vi "Autonomous selections.vi"() -> (3 "Autonomous selections":string[](array[string]))   [LabVIEW 2015]
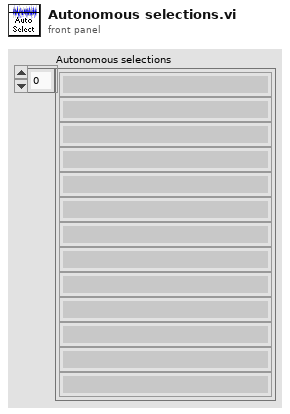
[diagram p1: front panel]
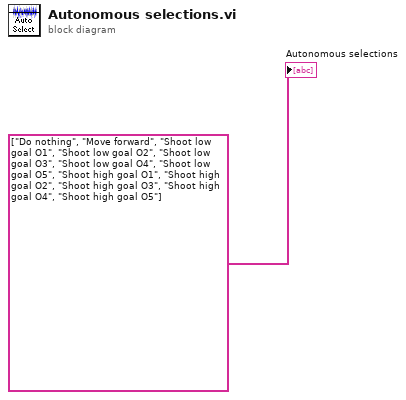
[diagram p0: block diagram]
diagram:
  "Autonomous selections" <- string[] ["Do nothing", "Move forward", "Shoot low goal O1", "Shoot low goal O2", "Shoot low goal O3", "Shoot low goal O4", "Shoot low goal O5", "Shoot high goal O1", "Shoot high goal O2", "Shoot high goal O3", "Shoot high goal O4", "Shoot high goal O5"] ("String Array")
